vi "SelectMeasurement.vi"(8 "error in (no error)":errorcluster, 9 "Meas Name":string="MY_MEAS", 10 "Channel":u32=1, 11 "resource name":refnum<k15>) -> (0 "error out":errorcluster)   [LabVIEW 2014]
doc: "Sets the selected measurement."
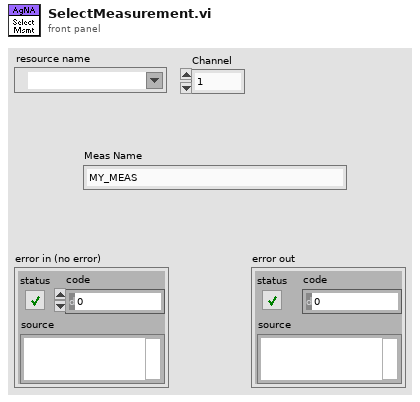
[diagram p1: front panel]
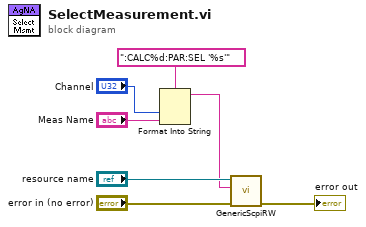
[diagram p0: block diagram]
diagram:
  n1 = Format Into String(format string=":CALC%d:PAR:SEL '%s'" ("Channel"), "Channel", "Meas Name") -> (resulting string=w4:string)  [unwired: 2 in, 1 out]
  n2 = call "GenericScpiRW.vi"("error in (no error)"="error in (no error)", "SCPI Command"=w4, "resource name"="resource name") -> ("error out"=→"error out":errorcluster)  [unwired: 7 in, 1 out]
